vi "Auto_Routine_DepositBalance.vi"(8 "error in (no error)":errorcluster) -> (0 "error out":errorcluster)   [LabVIEW 2020]
doc: "Deposites a cone on the upper node then balances\nInputs:\n--ErrorIn--\nOutputs:\n--ErrorOut--"
uses:
  Arm/ArmPositionPreset.ctl
  Arm/ArmGamePiecePreset.ctl
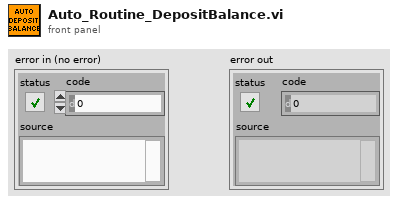
[diagram p1: front panel]
types:
  T1 = typedef "ArmGamePiecePreset.ctl" = enum16{"Cube", "Cone"}
  T2 = typedef "ArmPositionPreset.ctl" = enum16{"Upper", "Lower", "Middle", "Shelf", "Floor"}
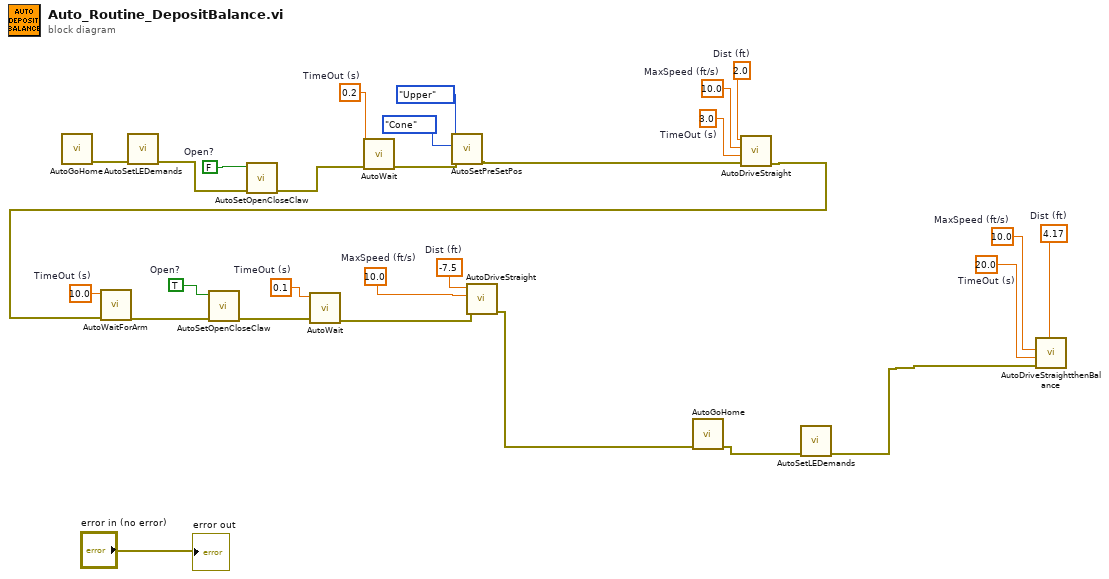
[diagram p0: block diagram]
diagram:
  w24 = 20.0  # TimeOut (s)
  w23 = 4.17  # Dist (ft)
  w22 = 10.0  # MaxSpeed (ft/s)
  w21 = 10.0  # MaxSpeed (ft/s)
  w28 = 3.0  # TimeOut (s)
  w27 = 10.0  # MaxSpeed (ft/s)
  w26 = 2.0  # Dist (ft)
  w19 = -7.5  # Dist (ft)
  w18 = 0.1  # TimeOut (s)
  w16 = TRUE  # Open?
  w14 = 10.0  # TimeOut (s)
  w11 = 0.2  # TimeOut (s)
  w10 = FALSE  # Open?
  n1 = call "AutoGoHome.vi"() -> ("error out"=w1:errorcluster)  [unwired: 11 in]
  n2 = call "AutoSetLEDemands.vi"("error in (no error)"=w1) -> ("error out"=w13:errorcluster)  [unwired: 10 in]
  n3 = call "AutoSetOpenCloseClaw.vi"("error in (no error)"=w13, "Open?"=w10) -> ("error out"=w6:errorcluster)  [unwired: 9 in]
  n4 = call "AutoWait.vi"("error in (no error)"=w6, "TimeOut (s)"=w11) -> ("error out"=w12:errorcluster)  [unwired: 9 in]
  n5 = call "AutoSetPreSetPos.vi"("error in (no error)"=w12, "Game Piece"=ArmGamePiecePreset."Cone", "Position"=ArmPositionPreset."Upper") -> ("error out"=w4:errorcluster)  [unwired: 8 in]
  n6 = call "AutoDriveStraight.vi"("error in (no error)"=w4, "TimeOut (s)"=w28, "MaxSpeed (ft/s)"=w27, "Dist (ft)"=w26) -> ("error out"=w25:errorcluster)  [unwired: 7 in]
  n7 = call "AutoWaitForArm.vi"("error in (no error)"=w25, "TimeOut (s)"=w14) -> ("error out"=w15:errorcluster)  [unwired: 9 in]
  n8 = call "AutoSetOpenCloseClaw.vi"("error in (no error)"=w15, "Open?"=w16) -> ("error out"=w17:errorcluster)  [unwired: 9 in]
  n9 = call "AutoWait.vi"("error in (no error)"=w17, "TimeOut (s)"=w18) -> ("error out"=w20:errorcluster)  [unwired: 9 in]
  n10 = call "AutoDriveStraight.vi"("error in (no error)"=w20, "MaxSpeed (ft/s)"=w21, "Dist (ft)"=w19) -> ("error out"=w2:errorcluster)  [unwired: 8 in]
  n11 = call "AutoGoHome.vi"("error in (no error)"=w2) -> ("error out"=w3:errorcluster)  [unwired: 10 in]
  n12 = call "AutoSetLEDemands.vi"("error in (no error)"=w3) -> ("error out"=w5:errorcluster)  [unwired: 10 in]
  n13 = call "AutoDriveStraightthenBalance.vi"("error in (no error)"=w5, "TimeOut (s)"=w24, "MaxSpeed (ft/s)"=w22, "Dist (ft)"=w23) -> ()  [unwired: 7 in, 1 out]
  "error out" <- "error in (no error)"
